vi "Specify Delete Action.vi"(11 "Platform Application in":refnum<class "Platform Application.lvclass">) -> (2 "Delete action":string, 3 "Platform Application out":refnum<class "Platform Application.lvclass">)   [LabVIEW 2015, in "NI_AWS_SNS.lvlib" / "Platform Application.lvclass"]
uses:
  Platform Application.lvclass
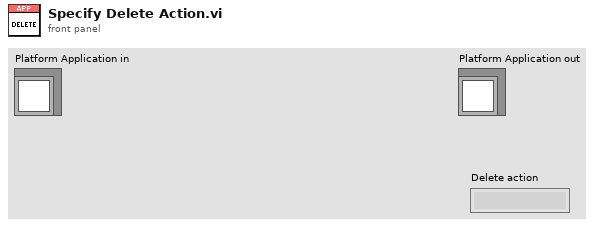
[diagram p1: front panel]
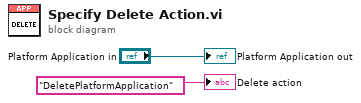
[diagram p0: block diagram]
diagram:
  "Platform Application out" <- "Platform Application in"
  "Delete action" <- "DeletePlatformApplication" ("value")
